vi "LB_FocusIndex_Tests.vi"(11 "error in":errorcluster) -> (15 "error out":errorcluster)   [LabVIEW 2016, in "DronaTest.lvlib"]
uses:
  DronaTest.lvlib
  APIs/Stimulus/ControlValue/SetValueAuto.vi
  APIs/Stimulus/ControlValue/Controls/Listbox/SetValueByItemIndex.vi
  APIs/Assert/AssertControlValue/Controls/Listbox/AssertValueByFocusIndex.vi
  <vilib>/addons/_JKI Toolkits/Caraya/classes/Assert/Assert Error.vi
  <vilib>/addons/_JKI Toolkits/Caraya/classes/Assert/Assert Equal Value_Variant.vi
  <vilib>/addons/_JKI Toolkits/Caraya/classes/Test/Test.lvclass
  Drona.lvlib
  <vilib>/SLL Toolkit/SLL Debug/SLL Debug.lvlib
  APIs/Stimulus/ControlValue/Controls/Listbox/StimulusListbox.lvlib
  APIs/Stimulus/ControlValue/ControlValue.lvlib
  <vilib>/addons/_JKI Toolkits/Caraya/classes/Assert/Assert.lvclass
  APIs/Assert/AssertControlValue/Controls/Listbox/AssertListbox.lvlib
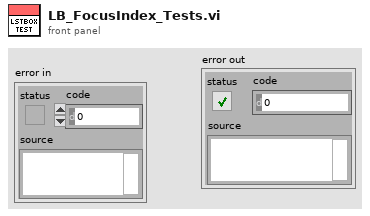
[diagram p1: front panel]
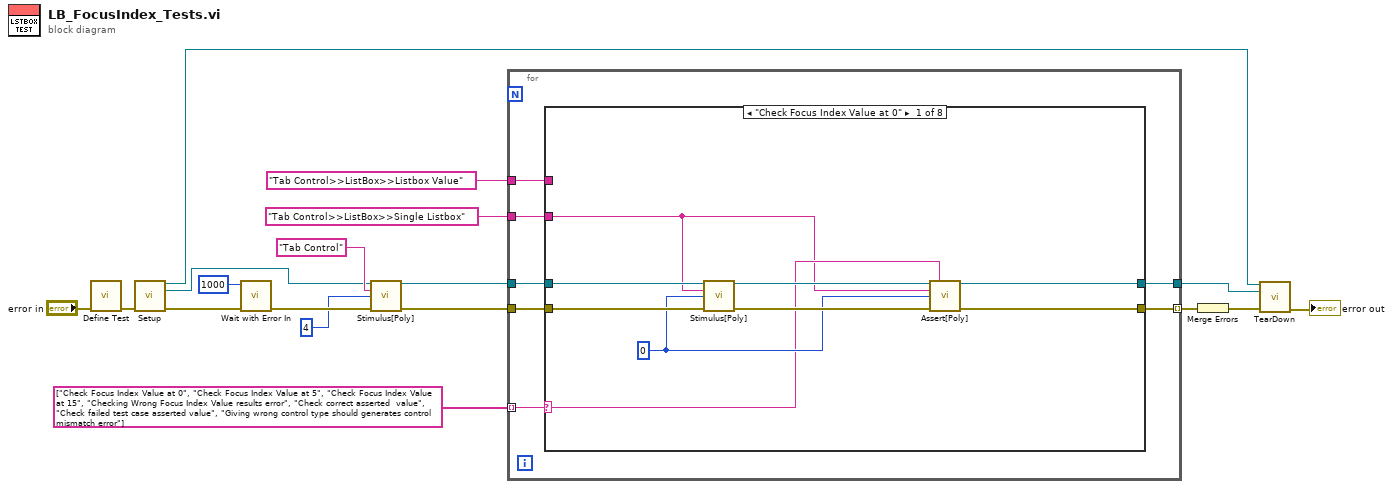
[diagram p0: block diagram]
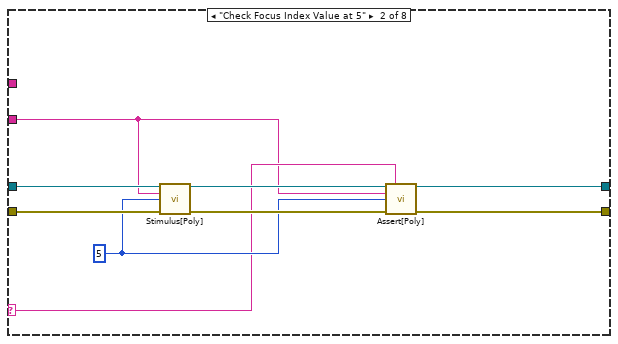
[diagram p2: hidden frame]
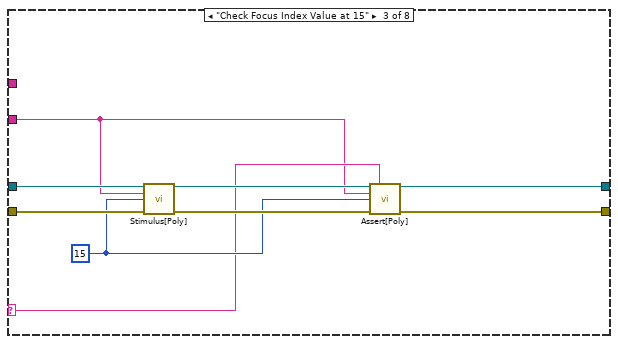
[diagram p3: hidden frame]
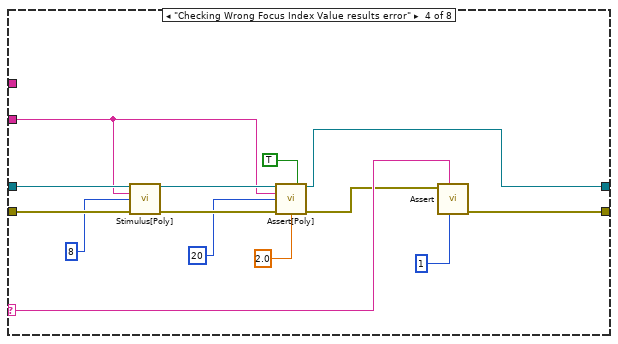
[diagram p4: hidden frame]
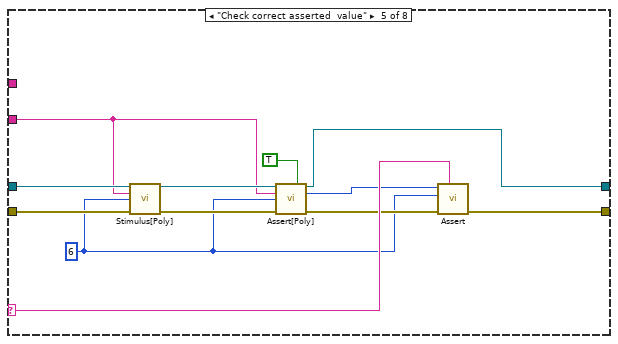
[diagram p5: hidden frame]
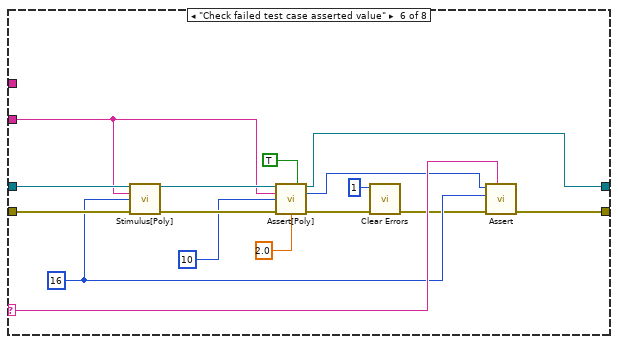
[diagram p6: hidden frame]
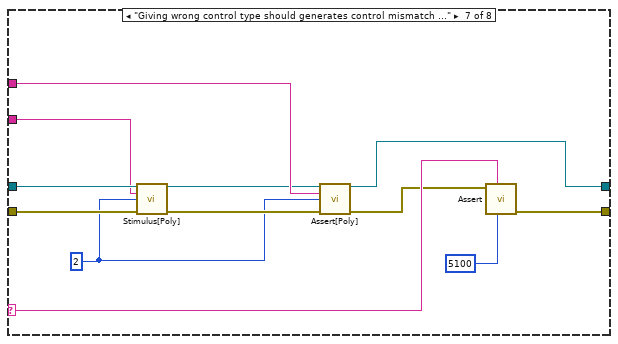
[diagram p7: hidden frame]
diagram:
  n1 = call <vilib>:"Define Test.vi"("error in (no error)"="error in") -> ("error out"=w7:errorcluster)  [unwired: 9 in, 1 out]
  n2 = call "Setup.vi"("error in (no error)"=w7) -> ("Application Ref"=w3:refnum<vi>, "VI out"=w5:refnum<vi>, "error out"=w6:errorcluster)  [unwired: 12 in]
  n3 = call <vilib>:"Wait with Error In.vi"("error in (no error)"=w6, "milliseconds to wait"=u32 1000) -> ("error out"=w16:errorcluster)  [unwired: 9 in]
  n4 = call-poly "Stimulus[Poly].vi"("VI Reference In"=w5, "Control Path"="Tab Control", "Value (Signaling)"=4, "error in"=w16) -> ("VI Reference Out"=w12:refnum<vi>, "error out"=w15:errorcluster)  [unwired: 10 in]
  n5 = for {
    tunnel: w12 -> [w24]
    tunnel: "Tab Control>>ListBox>>Single Listbox" ("Control Path") -> [w23]
    tunnel: "Tab Control>>ListBox>>Listbox Value" ("Control Path") -> [w22]
    tunnel: string[] ["Check Focus Index Value at 0", "Check Focus Index Value at 5", "Check Focus Index Value at 15", "Checking Wrong Focus Index Value results error", "Check correct asserted  value", "Check failed test case asserted value", "Giving wrong control type should generates control mismatch error"] -> [w20] mode=indexing
    tunnel: [w19] -> w2
    tunnel: w15 -> [w25]
    tunnel: [w21] -> w8 mode=indexing
    n6 = case shown="\"Check Focus Index Value at 0\"" w20 {
      selector: w20 -> [w27 w36 w45 w65 w77 w93 w105 _]
      tunnel: w25 -> [w34 w43 w52 w63 w76 w92 w100 w108]
      tunnel: w24 -> [w33 w42 w51 w62 w75 w91 w98 w107]
      tunnel: w23 -> [w26 w35 w44 w58 w72 w88 w96 _]
      tunnel: w22 -> [_ _ _ _ _ _ w102 _]
      tunnel: [w29 w38 w47 w66 w78 w94 w106 w108] -> w21
      tunnel: [w28 w37 w46 w56 w71 w87 w101 w107] -> w19
      frame "Check Focus Index Value at 0" {
        w30 = 0 ("Item Index")
        n7 = call-poly "Stimulus[Poly].vi"("VI Reference In"=w33, "Control Path"=w26, "Item Index"=w30, "Error In"=w34) -> ("VI Reference Out"=w31:refnum<vi>, "Error Out"=w32:errorcluster)  [unwired: 10 in]
        n8 = call-poly "Assert[Poly].vi"("VI Reference In"=w31, "Test Label"=w27, "Control Path"=w26, "Focus Index"=w30, "Error In"=w32) -> ("VI Reference Out"=w28:refnum<vi>, "Error Out"=w29:errorcluster)  [unwired: 8 in, 1 out]
      }
      frame "Check Focus Index Value at 5" {
        w39 = 5 ("Item Index")
        n9 = call-poly "Stimulus[Poly].vi"("VI Reference In"=w42, "Control Path"=w35, "Item Index"=w39, "Error In"=w43) -> ("VI Reference Out"=w40:refnum<vi>, "Error Out"=w41:errorcluster)  [unwired: 10 in]
        n10 = call-poly "Assert[Poly].vi"("VI Reference In"=w40, "Test Label"=w36, "Control Path"=w35, "Focus Index"=w39, "Error In"=w41) -> ("VI Reference Out"=w37:refnum<vi>, "Error Out"=w38:errorcluster)  [unwired: 8 in, 1 out]
      }
      frame "Check Focus Index Value at 15" {
        w48 = 15 ("Item Index")
        n11 = call-poly "Stimulus[Poly].vi"("VI Reference In"=w51, "Control Path"=w44, "Item Index"=w48, "Error In"=w52) -> ("VI Reference Out"=w49:refnum<vi>, "Error Out"=w50:errorcluster)  [unwired: 10 in]
        n12 = call-poly "Assert[Poly].vi"("VI Reference In"=w49, "Test Label"=w45, "Control Path"=w44, "Focus Index"=w48, "Error In"=w50) -> ("VI Reference Out"=w46:refnum<vi>, "Error Out"=w47:errorcluster)  [unwired: 8 in, 1 out]
      }
      frame "Checking Wrong Focus Index Value results error" {
        n13 = call-poly "Stimulus[Poly].vi"("VI Reference In"=w62, "Control Path"=w58, "Item Index"=8, "Error In"=w63) -> ("VI Reference Out"=w59:refnum<vi>, "Error Out"=w60:errorcluster)  [unwired: 10 in]
        n14 = call-poly "Assert[Poly].vi"("VI Reference In"=w59, "Assert Only? (F)"=TRUE, "Control Path"=w58, "Focus Index"=20 ("Item Index"), "Error In"=w60, "Timeout(5 sec)"=2.0) -> ("VI Reference Out"=w56:refnum<vi>, "Error Out"=w55:errorcluster)  [unwired: 7 in, 1 out]
        n15 = call-poly <vilib>:"Assert.vi"("error code (1)"=1, "Label"=w65, "Error?"=w55) -> ("error out"=w66:errorcluster)  [unwired: 7 in, 1 out]
      }
      frame "Check correct asserted  value" {
        w68 = 6 ("Item Index")
        n16 = call-poly "Stimulus[Poly].vi"("VI Reference In"=w75, "Control Path"=w72, "Item Index"=w68, "Error In"=w76) -> ("VI Reference Out"=w73:refnum<vi>, "Error Out"=w74:errorcluster)  [unwired: 10 in]
        n17 = call-poly "Assert[Poly].vi"("VI Reference In"=w73, "Assert Only? (F)"=TRUE, "Control Path"=w72, "Focus Index"=w68, "Error In"=w74) -> ("VI Reference Out"=w71:refnum<vi>, "Asserted Value"=w69:i32, "Error Out"=w70:errorcluster)  [unwired: 8 in]
        n18 = call-poly <vilib>:"Assert.vi"("Label"=w77, "error in (no error)"=w70, "Y"=w68, "X"=w69) -> ("error out"=w78:errorcluster)  [unwired: 6 in, 1 out]
      }
      frame "Check failed test case asserted value" {
        w85 = 16 ("Item Index")
        n19 = call-poly "Stimulus[Poly].vi"("VI Reference In"=w91, "Control Path"=w88, "Item Index"=w85, "Error In"=w92) -> ("VI Reference Out"=w89:refnum<vi>, "Error Out"=w90:errorcluster)  [unwired: 10 in]
        n20 = call-poly "Assert[Poly].vi"("VI Reference In"=w89, "Assert Only? (F)"=TRUE, "Control Path"=w88, "Focus Index"=10 ("Item Index"), "Error In"=w90, "Timeout(5 sec)"=2.0) -> ("VI Reference Out"=w87:refnum<vi>, "Asserted Value"=w79:i32, "Error Out"=w86:errorcluster)  [unwired: 7 in]
        n21 = call <vilib>:"Clear Errors.vi"("error in (no error)"=w86, "specific error code to clear (0: all)"=1) -> ("error out"=w81:errorcluster)  [unwired: 4 in, 1 out]
        n22 = call-poly <vilib>:"Assert.vi"("Label"=w93, "error in (no error)"=w81, "Y"=w85, "X"=w79) -> ("error out"=w94:errorcluster)  [unwired: 6 in, 1 out]
      }
      frame "Giving wrong control type should generates control mismatch error" {
        w95 = 2 ("Item Index")
        n23 = call-poly "Stimulus[Poly].vi"("VI Reference In"=w98, "Control Path"=w96, "Item Index"=w95, "Error In"=w100) -> ("VI Reference Out"=w97:refnum<vi>, "Error Out"=w99:errorcluster)  [unwired: 10 in]
        n24 = call-poly "Assert[Poly].vi"("VI Reference In"=w97, "Control Path"=w102, "Focus Index"=w95, "Error In"=w99) -> ("VI Reference Out"=w101:refnum<vi>, "Error Out"=w103:errorcluster)  [unwired: 9 in, 1 out]
        n25 = call-poly <vilib>:"Assert.vi"("error code (1)"=5100, "Label"=w105, "Error?"=w103) -> ("error out"=w106:errorcluster)  [unwired: 7 in, 1 out]
      }
      frame Default {
      }
    }
  }
  n26 = Merge Errors(w8) -> (w4:errorcluster)
  n27 = call "TearDown.vi"("Application Ref"=w3, "VI in"=w2, "error in (no error)"=w4) -> ("error out"=→"error out":errorcluster)  [unwired: 12 in]
